vi "Transfer Immediate_wrapper.vi"() -> ()   [LabVIEW 2025]
uses:
  <vilib>/Rock Robotics/WPI/Framework/Command Status Info.ctl
  <vilib>/Rock Robotics/WPI/Framework/Completion Status.ctl
  <vilib>/Rock Robotics/WPI/Framework/Completion Notifier.ctl
  Implementation/Transfer Operations.ctl
panel:
  in  "Operation":T1
  out "Command Info Out":T2
  in  "Setpoint":dbl
  in  "Command Info In":T2
  in  "Description":string
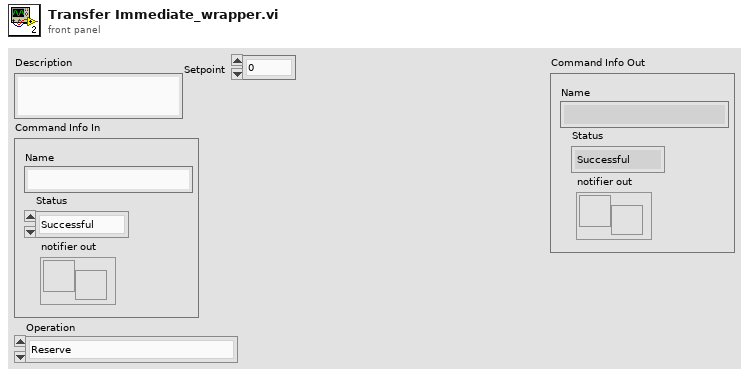
[diagram p1: front panel]
types:
  T1 = typedef "Transfer Operations.ctl" = enum16{"Reserve", "Read Current", "Immediate", "Start Transfer"}
  T2 = typedef "Command Status Info.ctl" = cluster{"Name":string, "Status":T3, "notifier out":T4}
  T3 = typedef "Completion Status.ctl" = enum16{"Successful", "Aborted", "Incomplete"}
  T4 = typedef "Completion Notifier.ctl" = refnum<notifier>
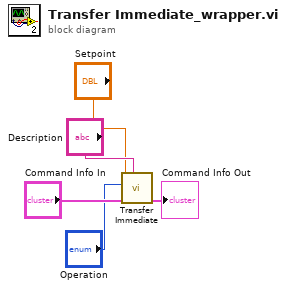
[diagram p0: block diagram]
diagram:
  n1 = call "Transfer Immediate.vi"("Description"="Description", "Command Info In"="Command Info In", "Operation"="Operation", "Setpoint"="Setpoint") -> ("Command Info Out"=→"Command Info Out":T2)  [unwired: 7 in]
